vi "Index_Logic.vi"(0 "X":bool, 4 "Intake Pressed":bool, 6 "B":bool, 7 "Right Trigger":dbl, 8 "Y":bool, 9 "A":bool, 10 "Reject Pressed":bool, 11 "Elevate Pressed":bool) -> ()   [LabVIEW 2020]
uses:
  <vilib>/Rock Robotics/WPI/ThirdParty/Phoenix-LabVIEW/Motor Controller/Controls/CTRE_Phoenix_MotorControl_ControlMode.ctl
  <vilib>/Rock Robotics/WPI/Solenoid/WPI_SolenoidValue.ctl
  <vilib>/Rock Robotics/Network Tables/NT Read String.vi
  <vilib>/Rock Robotics/Network Tables/NT Write Boolean.vi
  <vilib>/Rock Robotics/WPI/Solenoid/WPI_SolenoidSetEnum.vi
panel:
  in  "Intake want":dbl=0.75
  in  "Elevate want":dbl=-0.35
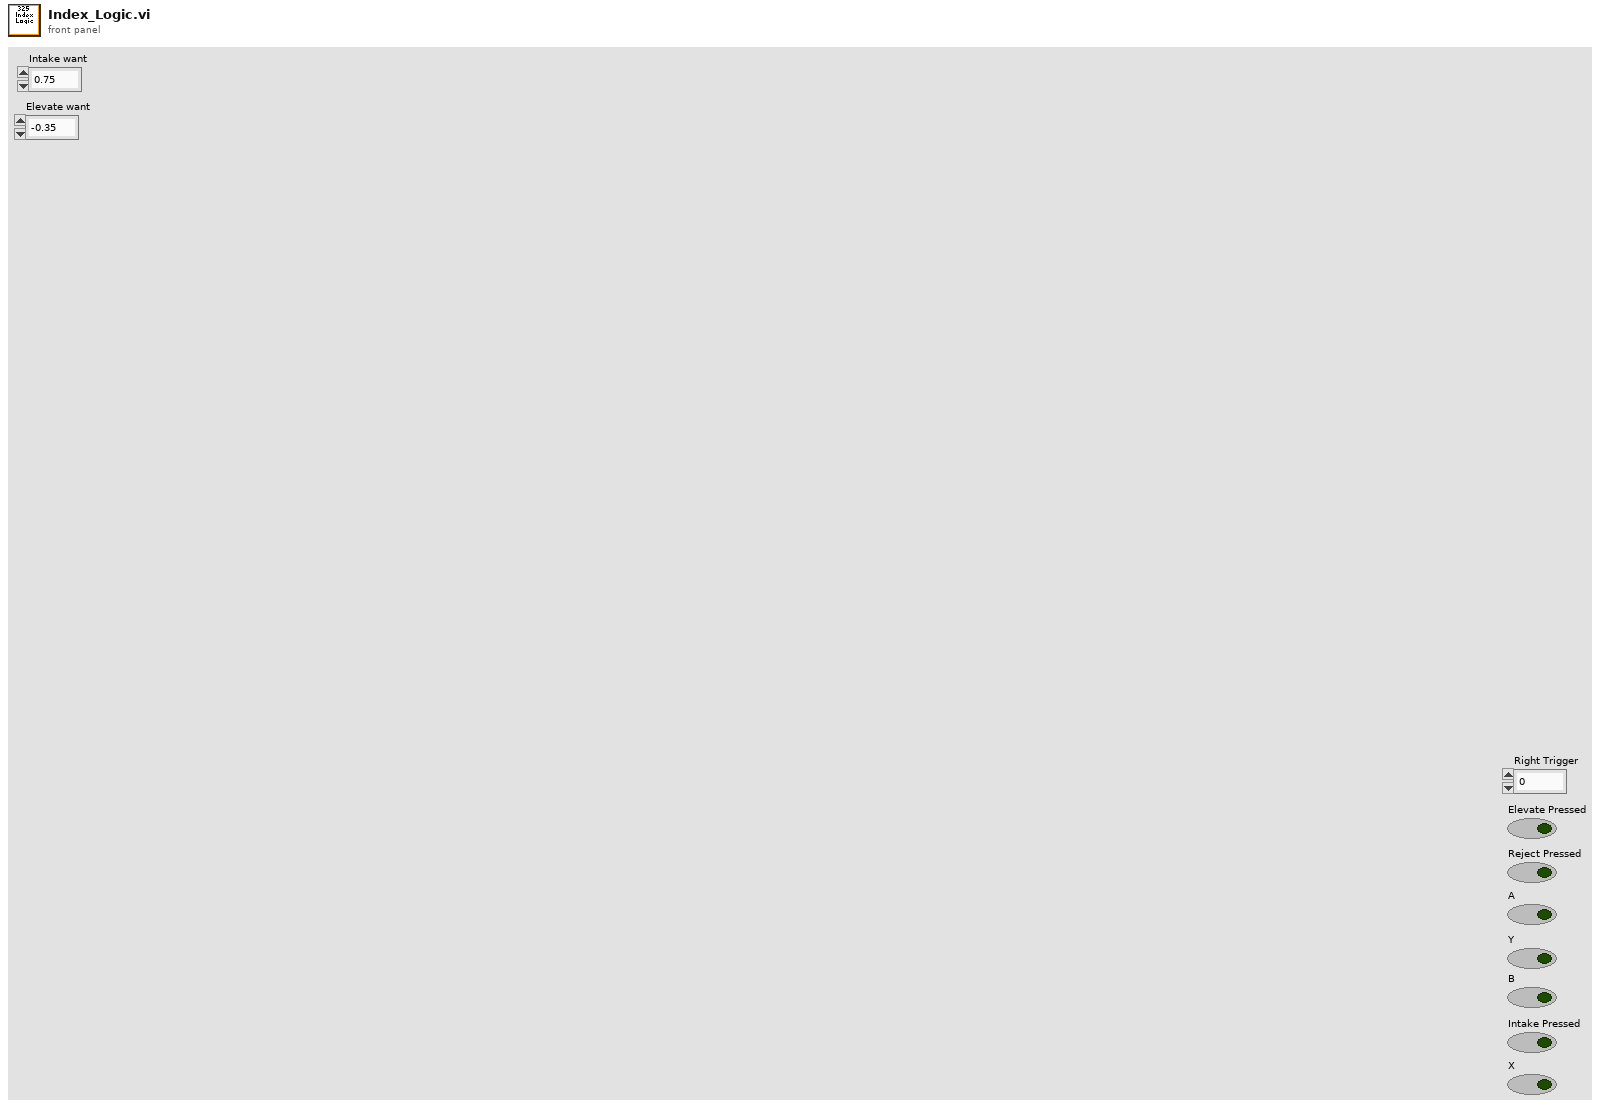
[diagram p1: front panel]
types:
  T1 = typedef "CTRE_Phoenix_MotorControl_ControlMode.ctl" = u16
  T2 = typedef "WPI_SolenoidValue.ctl" = enum16{"Off", "On", "Forward", "Reverse"}
  T3 = typedef "WPI_SolenoidDevRef.ctl" = cluster{"DevStatus":errorcluster, "Pneumatics Control Module":u8, "Forward Solenoid Channel":T4, "Reverse Solenoid Channel":T4}
  T4 = typedef "WPI_SolenoidChannel.ctl" = enum8{"Solenoid 0", "Solenoid 1", "Solenoid 2", "Solenoid 3", "Solenoid 4", "Solenoid 5", "Solenoid 6", "Solenoid 7", "Solenoid 8", "Solenoid 9", "Solenoid 10", "Solenoid 11", "Solenoid 12", "Solenoid 13", "Solenoid 14", "Solenoid 15", "Invalid"}
  T5 = typedef "WPI_MotorControlDeviceRef.ctl" = cluster{"DeviceStatus":errorcluster, "Type":T6, "PWM":cluster{"PWM Channel":T7, "DeadBand":T8}, "CAN":cluster{"Device Number":u8, "SetOutput VI Ref":variant, "GetOutput VI Ref":variant, "Enable VI Ref":variant, "Disable VI Ref":variant, "Data":variant}, "Invert":bool, "DIO PWM":cluster{"PWM \"Enable\" Channel":T7, "DIOChannel":T9, "PWM Rate":dbl}}
  T6 = typedef "WPI_MotorControlType.ctl" = enum16{"PWM", "CAN", "DIO PWM"}
  T7 = typedef "FPGA_DIOPWMChannel.ctl" = enum8{"PWM 0", "PWM 1", "PWM 2", "PWM 3", "PWM 4", "PWM 5", "PWM 6", "PWM 7", "PWM 8", "PWM 9", "PWM MXP 0", "PWM MXP 1", "PWM MXP 2", "PWM MXP 3", "PWM MXP 4", "PWM MXP 5", "PWM MXP 6", "PWM MXP 7", "PWM MXP 8", "PWM MXP 9", "Invalid"}
  T8 = typedef "WPI_PWMDeadband.ctl" = cluster{"Name":string, "maxPositivePwm":i32, "minPositivePwm":i32, "centerPwm":i32, "maxNegativePwm":i32, "minNegativePwm":i32, "angularRange":u16}
  T9 = typedef "FPGA_DIOChannel.ctl" = enum8{"DIO 0", "DIO 1", "DIO 2", "DIO 3", "DIO 4", "DIO 5", "DIO 6", "DIO 7", "DIO 8", "DIO 9", "DIO MXP 0", "DIO MXP 1", "DIO MXP 2", "DIO MXP 3", "DIO MXP 4", "DIO MXP 5", "DIO MXP 6", "DIO MXP 7", "DIO MXP 8", "DIO MXP 9", "DIO MXP 10", "DIO MXP 11", "DIO MXP 12", "DIO MXP 13", "DIO MXP 14", "DIO MXP 15", "SPI Port CS1", "SPI Port CS2", "SPI Port CS3", "SPI Port MISO", "SPI Port MOSI", "Invalid"}
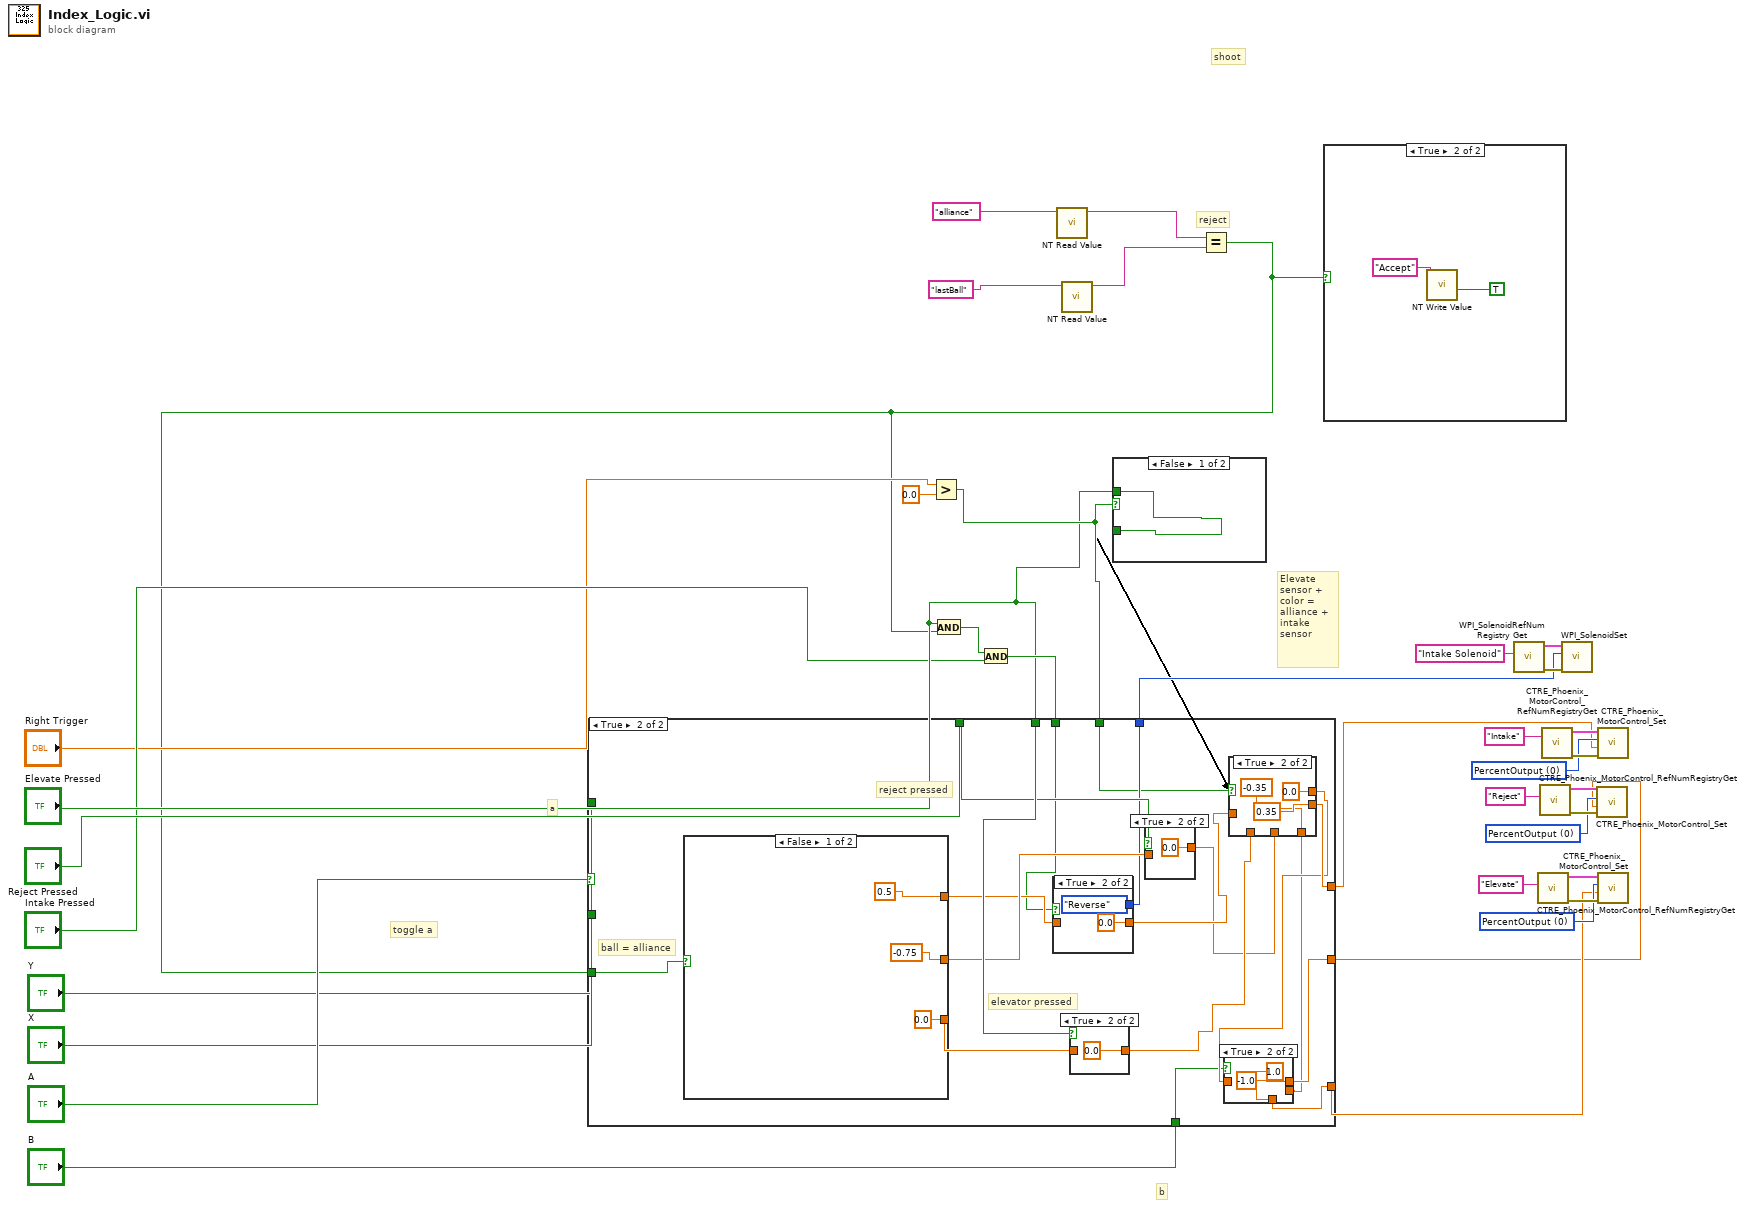
[diagram p0: block diagram]
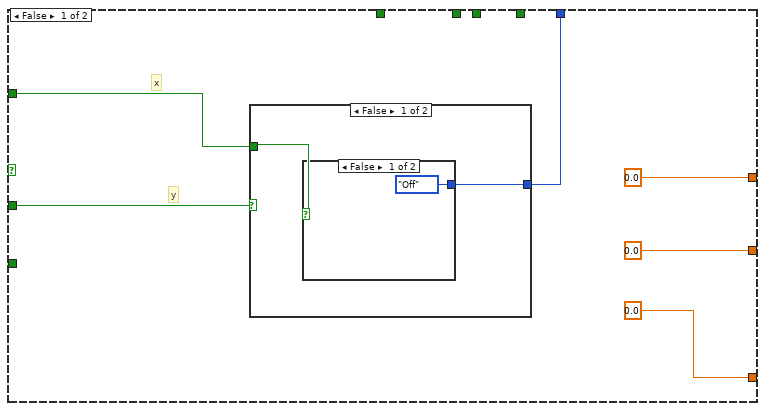
[diagram p2: hidden frame]
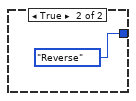
[diagram p3: hidden frame]
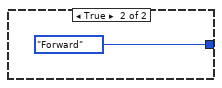
[diagram p4: hidden frame]
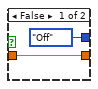
[diagram p7: hidden frame]
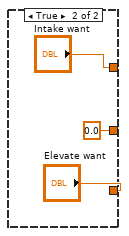
[diagram p10: hidden frame]
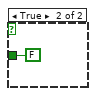
[diagram p11: hidden frame]
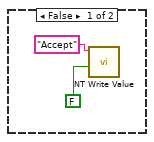
[diagram p12: hidden frame]
diagram:
  w25 = T1 0 items=["PercentOutput"=0, "Position"=1, "Velocity"=2, "Current"=3, "Follower"=5, "MotionProfile"=6, "MotionMagic"=7, "MotionProfileArc"=10, "Disabled"=15] ("Control Mode")
  w26 = T1 0 items=["PercentOutput"=0, "Position"=1, "Velocity"=2, "Current"=3, "Follower"=5, "MotionProfile"=6, "MotionMagic"=7, "MotionProfileArc"=10, "Disabled"=15] ("Control Mode")
  w27 = T1 0 items=["PercentOutput"=0, "Position"=1, "Velocity"=2, "Current"=3, "Follower"=5, "MotionProfile"=6, "MotionMagic"=7, "MotionProfileArc"=10, "Disabled"=15] ("Control Mode")
  # "toggle a"
  # "Elevate sensor + color = alliance + intake sensor"
  # "b"
  # "a"
  # "shoot"
  # "reject"
  n1 = Greater?(x="Right Trigger", y=0.0) -> (0:w10:bool)
  n2 = call-poly <vilib>:"NT Read Value.vi"("Name"="alliance") -> ("String"=w24:string)  [unwired: 9 in, 1 out]
  n3 = call-poly <vilib>:"NT Read Value.vi"("Name"="lastBall") -> ("String"=w21:string)  [unwired: 9 in, 1 out]
  n4 = case shown="False" w10 {
    tunnel: "Elevate Pressed" -> [w37 _]
    tunnel: [w37 FALSE ("Switch Pressed")] -> _
    frame False {
    }
    frame True {
    }
  }
  n5 = Equal?(x=w24, y=w21) -> (x = y?=w1:bool)
  n6 = And(x="Elevate Pressed", y=w1) -> (x .and. y?=w14:bool)
  n7 = And(x=w14, y="Intake Pressed") -> (x .and. y?=w13:bool)
  n8 = case shown="True" "A" {
    tunnel: w1 -> [_ w67]
    tunnel: [0.0 ("Intake want") w59] -> w16
    tunnel: [0.0 ("Elevate 1") w51] -> w17
    tunnel: "Elevate Pressed" -> [_ w66]
    tunnel: [0.0 ("Reject no want") w54] -> w15
    tunnel: "Reject Pressed" -> [_ w64]
    tunnel: w13 -> [_ w50]
    tunnel: [w41 w61] -> w12
    tunnel: w10 -> [_ w57]
    tunnel: "B" -> [_ w53]
    tunnel: "Y" -> [w40 _]
    tunnel: "X" -> [w39 _]
    frame False {
      # "x"
      # "y"
      n9 = case shown="False" w40 {
        tunnel: [w46 WPI_SolenoidValue."Forward" ("Value")] -> w41
        tunnel: w39 -> [w45 _]
        frame False {
          n10 = case shown="False" w45 {
            tunnel: [WPI_SolenoidValue."Off" ("Value") WPI_SolenoidValue."Reverse" ("Value")] -> w46
            frame False {
            }
            frame True {
            }
          }
        }
        frame True {
        }
      }
    }
    frame True {
      # "reject pressed"
      # "elevator pressed"
      # "ball = alliance"
      n11 = case shown="False" w67 {
        tunnel: [0.0 ("Elevate want") "Elevate want"] -> w65
        tunnel: [0.5 ("Intake 1") "Intake want"] -> w62
        tunnel: [-0.75 ("Reject no want") 0.0 ("Reject no want")] -> w63
        frame False {
        }
        frame True {
        }
      }
      n12 = case shown="True" w50 {
        tunnel: w62 -> [w79 _]
        tunnel: [w79 0.0 ("Intake want")] -> w60
        tunnel: [WPI_SolenoidValue."Off" ("Value") WPI_SolenoidValue."Reverse" ("Value")] -> w61
        frame False {
        }
        frame True {
        }
      }
      n13 = case shown="True" w66 {
        tunnel: [w84 0.0 ("Elevate 1")] -> w58
        tunnel: w65 -> [w84 _]
        frame False {
        }
        frame True {
        }
      }
      n14 = case shown="True" w64 {
        tunnel: w63 -> [w82 _]
        tunnel: [w82 0.0 ("Reject no want")] -> w56
        frame False {
        }
        frame True {
        }
      }
      n15 = case shown="True" w57 {
        tunnel: w60 -> [w74 _]
        tunnel: [w74 0.35 ("Intake want")] -> w59
        tunnel: w58 -> [w73 _]
        tunnel: [w73 -0.35 ("Elevate 1")] -> w52
        tunnel: w56 -> [w72 _]
        tunnel: [w72 0.0 ("Reject no want")] -> w55
        frame False {
        }
        frame True {
        }
      }
      n16 = case shown="True" w53 {
        tunnel: w55 -> [w69 _]
        tunnel: [w69 -1.0 ("Reject no want")] -> w54
        tunnel: w52 -> [w68 _]
        tunnel: [w68 1.0 ("Elevate 1")] -> w51
        frame False {
        }
        frame True {
        }
      }
    }
  }
  n17 = case shown="True" w1 {
    frame False {
      n18 = call-poly <vilib>:"NT Write Value.vi"("Boolean"=FALSE, "Name"="Accept") -> ()  [unwired: 9 in, 1 out]
    }
    frame True {
      n19 = call-poly <vilib>:"NT Write Value.vi"("Boolean"=TRUE, "Name"="Accept") -> ()  [unwired: 9 in, 1 out]
    }
  }
  n20 = call <vilib>:"WPI_SolenoidRefNum Registry Get.vi"("refnum name"="Intake Solenoid") -> ("error out"=w20:errorcluster, "SolenoidDevRef"=w19:T3)  [unwired: 9 in]
  n21 = call <vilib>:"CTRE_Phoenix_MotorControl_RefNumRegistryGet.vi"("refnum name"="Elevate") -> ("error out"=w32:errorcluster, "PhoenixMotorControlDevRef"=w31:T5)  [unwired: 9 in]
  n22 = call <vilib>:"CTRE_Phoenix_MotorControl_RefNumRegistryGet.vi"("refnum name"="Reject") -> ("error out"=w34:errorcluster, "PhoenixMotorControlDevRef"=w33:T5)  [unwired: 9 in]
  n23 = call <vilib>:"CTRE_Phoenix_MotorControl_RefNumRegistryGet.vi"("refnum name"="Intake") -> ("error out"=w36:errorcluster, "PhoenixMotorControlDevRef"=w35:T5)  [unwired: 9 in]
  n24 = call-poly <vilib>:"WPI_SolenoidSet.vi"("error in (no error)"=w20, "Value"=w12, "SolenoidDevRef"=w19) -> ()  [unwired: 7 in, 2 out]
  n25 = call <vilib>:"CTRE_Phoenix_MotorControl_Set.vi"("error in (no error)"=w34, "Output"=w15, "Control Mode"=w25, "PhoenixMotorControlDevRef"=w33) -> ()  [unwired: 6 in, 2 out]
  n26 = call <vilib>:"CTRE_Phoenix_MotorControl_Set.vi"("error in (no error)"=w36, "Output"=w16, "Control Mode"=w26, "PhoenixMotorControlDevRef"=w35) -> ()  [unwired: 6 in, 2 out]
  n27 = call <vilib>:"CTRE_Phoenix_MotorControl_Set.vi"("error in (no error)"=w32, "Output"=w17, "Control Mode"=w27, "PhoenixMotorControlDevRef"=w31) -> ()  [unwired: 6 in, 2 out]
